vi "Day 3 task 1.vi"() -> ()   [LabVIEW 2022 SP3]
uses:
  fe08b190-bd30-44fb-9682-f841e3017fd9.vi
  baedc93f-74fa-4a9a-802a-d6937c73f20c.vi
  0b9a60e8-a408-4365-8614-b25103b5fdd8.vi
  <vilib>/Comparison/Less/Less Functor/Less Functor.lvclass
panel:
  out "sum":u64
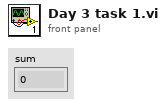
[diagram p1: front panel]
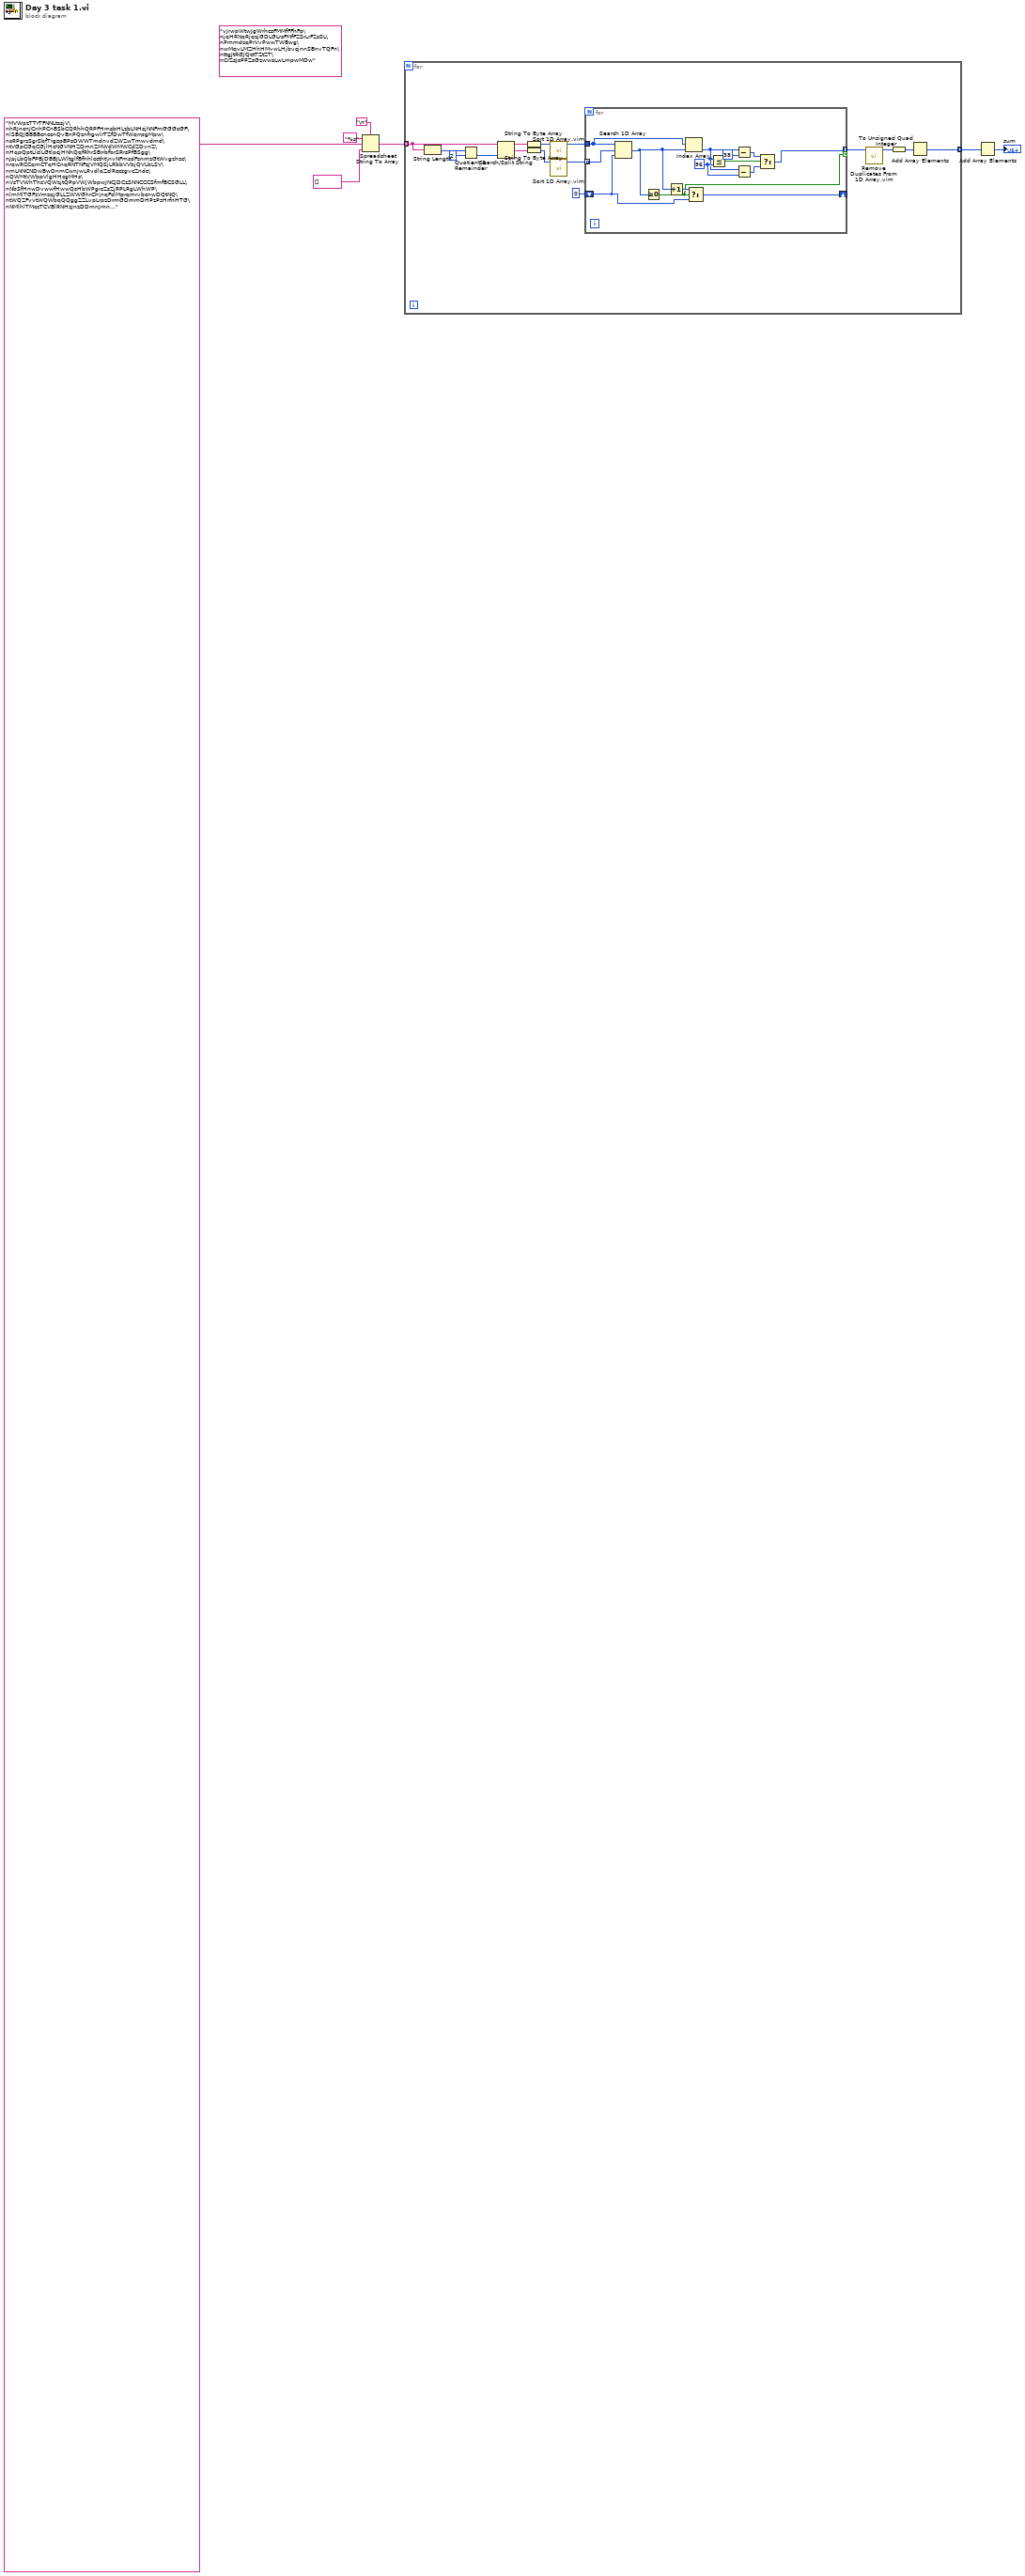
[diagram p0: block diagram]
diagram:
  (unwired) "vJrwpWtwJgWrhcsFMMfFFhFp\njqHRNqRjqzjGDLGLrsFMfFZSrLrFZsSL\nPmmdzqPrVvPwwTWBwg\nwMqvLMZHhHMvwLHjbvcjnnSBnvTQFn\nttgJtRGJQctTZtZT\nCrZsJsPPZsGzwwsLwLmpwMDw"
  n1 = Spreadsheet String To Array(delimiter (Tab)="\n", format string="%s", spreadsheet string="MVWpzTTrTFNNLtssjV\nhRJncnJCnhPCnBSbCQRhhQRPFHmsbHLzbLNHsjNNFmGGGsGF\nlSBQJBBBBcnccnQvBnPQznfrgwlrTZfDwTfWqrrpgMpw\nsRPgrzSgrSbfTrgspBPsDWWTmdnvdZWZwTmwvdmd\ntVGpCGqCGjlHcNGVNHZDmnZMWdWMWCdZDvnZ\nHqpQptLlclLGtlpcjHNhQqfRhrSBrrbfbrSRrsPfBSgg\nJpjLbQbFPBjDBBJLWltglfBfhhlcctht\nvNFmsdFsnmzGtWvgzhzc\nrqwRCCqmCTqHCnqRNTNFsJVMQSjLRbbVVbjQVLbLSV\nmLNNCNDwBwDnmCwnJwLRvdlqZclRccsgvcZndc\nQWMtVWbpVlgHHcgMHs\nVsTVWhThsVQWzjtQPpVWjWbpwJNCJDCzSNNCCCSfmfBCSGLL\nNbSfHnwDvwwfHwwQsHbWPgrsZsZjRPLRgLWhWP\nlmMlTGFzVmzqjGLLZWWGhrCh\nqFclMprqmrvbcnwDQtNQ\ntWQZFvvtWQWbqQQggZZLvpLrpzDrmGDmmDHPzPzHrfnHTG\nNMlhlTMccTCVBlRNHzJnzDDmnJmn...", array type (2D Dbl)=string[] [] ("format string")) -> (array=w3:string[])
  n2 = for {
    tunnel: w3 -> [w22] mode=indexing
    tunnel: [w9] -> w2 mode=indexing
    n3 = String Length(string=w22) -> (length=w21:i32)
    n4 = Quotient & Remainder(x=w21, y=2) -> (floor(x/y)=w20:i32)  [unwired: 1 out]
    n5 = Search/Split String(string=w22, offset (0)=w20) -> (substring before match=w18:string, match + rest of string=w17:string)  [unwired: 1 in, 1 out]
    n6 = String To Byte Array(string=w18) -> (unsigned byte array=w16:u8[])
    n7 = String To Byte Array(string=w17) -> (unsigned byte array=w15:u8[])
    n8 = call "Sort 1D Array.vim"("unsorted array"=w16) -> ("sorted array"=w14:u8[])  [unwired: 10 in]
    n9 = call "Sort 1D Array.vim"("unsorted array"=w15) -> ("sorted array"=w13:u8[])  [unwired: 10 in]
    n10 = for {
      tunnel: w14 -> [w34]
      tunnel: w13 -> [w36] mode=indexing
      shift-right: [w35] -> _
      shift-left: 0 -> [w31]
      tunnel: [w24] -> w11 mode=indexing if=w23
      w29 = u8 96 ("y")
      n11 = Search 1D Array(1D array=w34, element=w36, start index (0)=w31) -> (index of element=w33:i32)
      n12 = Greater Or Equal To 0?(x=w33) -> (x >= 0?=w23:bool)
      n13 = Increment(x=w33) -> (x+1=w32:i32)
      n14 = Index Array(array=w34, index=w33) -> (element=w27:u8)
      n15 = Select(t=w32, s=w23, f=w31) -> (s? t:f=w35:i32)
      n16 = Less Or Equal?(x=w27, y=w29) -> (x <= y?=w30:bool)
      n17 = Subtract(x=w27, y=u8 38) -> (x-y=w26:u8)
      n18 = Subtract(x=w27, y=w29) -> (x-y=w28:u8)
      n19 = Select(t=w26, s=w30, f=w28) -> (s? t:f=w24:u8)
    }
    n20 = call "Remove Duplicates From 1D Array.vim"("array"=w11) -> ("array with duplicates removed"=w10:u8[])  [unwired: 10 in]
    n21 = To Unsigned Quad Integer(1:w10) -> (0:w8:u64[])
    n22 = Add Array Elements(numeric array=w8) -> (sum=w9:u64)
  }
  n23 = Add Array Elements(numeric array=w2) -> (sum=→"sum":u64)
